vi "Magazine_Hardware_Globals.vi"() -> ()   [LabVIEW 2019]
panel:
  in  "Magazine_Vertical (BL)":string="Magazine_Vertical (BL)"
  in  "Magazine_Horizontal (BR)":string="Magazine_Horizontal (BR)"
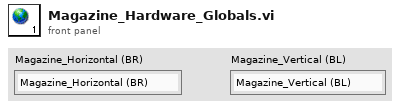
[diagram p1: front panel]
diagram:
